vi "AlliGator Send Plots to Image Profile Window.vi"(7 "Image Control Refnum":T2, 8 "error in (no error)":errorcluster, 9 "Fit Parameter":T1, 11 "AlliGator IV DVR in":refnum<data-value>) -> (0 "error out":errorcluster, 3 "AlliGator IV DVR out":refnum<data-value>)   [LabVIEW 2021, in "AlliGator Image Profile Window.lvlib"]
doc: "Computes plots and send them to the Profile Window."
uses:
  AlliGator Image Profile Window.lvlib
  AlliGator Internal Variables v2.ctl
  <vilib>/vision/Image Controls.llb/IMAQ Image.ctl
  AlliGator Gate Image Set.ctl
  AlliGator FLI Dataset Type.ctl
  AlliGator Data Series Type.ctl
  AlliGator Dataset Channel.ctl
  AlliGator Gate Arithmetic.ctl
  AlliGator Displayed Image.ctl
  Image/Named ROI Description.ctl
  AlliGator Decay Metadata v3.ctl
  AlliGator Decay Background Subtraction Info.ctl
  AlliGator Baseline Subtraction Method.ctl
  Graphs/XY Graph/XY Graph Plot Shift Parameters.ctl
  Graphs/XY Graph/XY Graph Plot Shift Method.ctl
  AlliGator Decay Extrapolation Parameters.ctl
  Phasor/Calibration Phasor (m, phi).ctl
  Phasor/Phasor Reference Series.ctl
  Phasor/Phasor Calibration Map v2.ctl
  Phasor/Phasor (g, s).ctl
  AlliGator Raw Phasor Plot Data v4.ctl
  Phasor/Phasor Standard Deviation Options.ctl
  AlliGator Phasor Multi-Harmonic Data.ctl
  Phasor/Phasor Harmonic Data.ctl
  AlliGator Decay Fit Options & Parameters v2.ctl
  Fits/IRF(X)PSED/Decay Fit Options v2.ctl
  Fits/Decay Convolution/Decay Model.ctl
  Fits/Residual Type.ctl
  Fits/IRF(X)PSED/Fit Weights Type.ctl
  Fits/Non-linear Fitting Method v2.ctl
  Fits/Fit Calculation Method.ctl
  Fits/Non-linear Fitting Algorithm.ctl
  AlliGator Decay Fit Parameter Constraints 2.ctl
  Fits/IRF(X)PSED/Decay Fit Parameters In List.ctl
  Fits/IRF(X)PSED/MLE Baseline Offset Type.ctl
  AlliGator Decay Preprocessing Parameters.ctl
  Fits/IRF(X)PSED/Decay Fit Parameters & Derived Quantities List.ctl
  Image/Image Control Refnum.ctl
  AlliGator Variables List.ctl
  AlliGator Source Image Profile Window Event Refnum.ctl
  AlliGator Image Profile Plot Data.ctl
  Graphs/XY Graph/XY Plot Data.ctl
  AlliGator Settings List.ctl
  Image/Box Profile Type.ctl
  AlliGator Image Profile Average Intensity Type.ctl
  AlliGator Image Profile Intensity Type.ctl
  Image/Image ROI Type.ctl
  Phasor/Phasor Ratio Type.ctl
  AlliGator Phasor Ratio Color-Coded Quantity.ctl
  Variant/Variant to Data/Variant to Boolean.vi
  Variant/Variant to Data/Variant to DBL.vi
  Variant/Variant to Data/Variant to U16.vi
  AlliGator Globals, Variables & Constants.lvlib
  Graphs/XY Graph/XY Graph Add-Ons.lvlib
  Image/Image.lvlib
  AlliGator Settings.lvlib
  Variant/Variant to Data/Variant to Data.lvlib
  AlliGator Decay Fit Parameter Map.lvlib
  Phasor/Phasor.lvlib
  AlliGator Phasor Ratio.lvlib
  Arrays/Arrays.lvlib
  Error/Error.lvlib
  AlliGator Internal Variables.lvlib
  AlliGator Files.lvlib
  AlliGator Phasor Graph.lvlib
  AlliGator Decay Preprocessing.lvlib
  AlliGator Phasor Plot.lvlib
  AlliGator Source Image.lvlib
  Fits/Fits.lvlib
  AlliGator Decay Fit.lvlib
  AlliGator Dual-Channel Datasets.lvlib
panel:
  # "see the AlliGator License on the block diagram (Ctrl+E or Window:Show Block Diagram)"
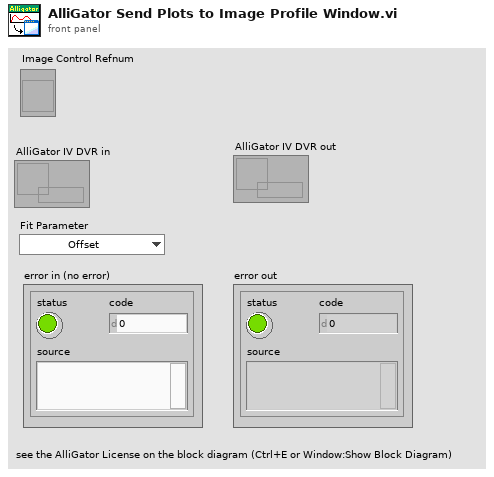
[diagram p1: front panel]
types:
  T1 = typedef "Fits.lvlib/Decay Fit Parameters & Derived Quantities List.ctl" = enum16{"Offset", "Baseline", "A_1", "tau_1", "A_2", "tau_2", "<tau>_a", "f1_a", "f2_a", "<tau>_i", "f1_i", "f2_i", "-", "R^2", "Chi^2"}
  T2 = typedef "Image.lvlib/Image Control Refnum.ctl" = refnum<vi>
  T3 = typedef "AlliGator Globals, Variables & Constants.lvlib/AlliGator Variables List.ctl" = enum16{"---- GUI ----", "Initialization Status", "State Indicators Refnum", "Original AlliGator Menu Items", "Current Action Loop State", "Script in progress", "Playback", "Loop Playback", "Search ROI Used", "Search ROI", "Decay Graph Max Legend Size", "Intensity Graph Max Legend Size", "Decay Statistics Graph Max Legend Size", "Phasor Graph Max Legend Size", "Phasor Ratio Graph Max Legend Size", "Lifetime Graph Max Legend Size", "---- Files ----", "Export Dataset Frames as Individual Files", "Show Batch Export Help Balloons", "Frames in Dataset", "ptu File Frame Start Indices", "Current Frame in Dataset", "Current Frame Timestamp", "------ Python Plugins ------", "Python Plugins Information", "Python Session", "Valid Python Session?", "---- Source Image ----", "Dataset Loaded", "Dataset Metadata", "Dataset Channel", "Dataset Data Description", "Background Dataset Metadata", "Background Dataset Channel", "Background Dataset Data Description", "Background File Subtraction", "Background File Path", "Background File Pile-up Correction", "Background File Pixel Well Capacity", "Background File Scaling Factor", "Source Image ROIs", "Current Source Image ROI", "Source Image ROI Event Refnum", "X_Source Image Display Range", "X_Source Image Palette Information", "Source Image Palette List", "Source Image Scale", "Current Dataset Load Settings", "Source Image:ROI Overlay Color", "---- Image Profile Window ----", "Image Profile:Overlay ROI in Source Image", "Image Profile Window Event Refnum", "Image Profile:IntensityType", "Image Profile:Intensity Average Type", "Image Profile:Intensity-weighted SDV", "Image Profile:Box Profile Type", "Image Profile Window Open", "Image Profile:Plotted Fit Parameter", "X_Type of Displayed Image", "X_Time Gate Slider", "Dataset Path", "Source Image Overlay to Erase", "Is Displayed Image Accumulated", "White Light Image Modified", "Mask Image Modified", "Macrotime Gate Separation", "------ Phasor Graph -------", "Phasor Graph:Show Line", "---- Phasor Plot ---", "Phasor Plot Parameters Changed", "FLI Dataset Modified since last Phasor Plot Calculation", "Phasor Harmonics Data", "Selected Phasor Harmonics", "Phasor Harmonic Manager Event Refnum", "Phasor Plot ROIs", "Current Phasor Plot ROI", "Phasor Plot ROI Event Refnum", "Phasor Plot Image Reference Points", "Phasor Plot Computed", "Phasor Plot Palette Information", "Phasor Plot Palette List", "Phasor Ratio Palette Information", "Phasor Ratio Palette List", "Phasor Image Scale", "Phasor Plot Image Overlay to Erase", "Phasor Plot Image Elements to Update", "Current Phasor Plot Calculation Parameters", "Current Phasor Calibration Options", "Reset Cumulated Phasor Plot", "Phasor Ratio Reference 1", "Phasor Ratio Lifetime Reference 1", "Phasor Ratio Reference 1 Frequency", "Phasor Ratio Reference 2", "Phasor Ratio Lifetime Reference 2", "Phasor Ratio Reference 2 Frequency", "---- Decay Analysis ----", "Number of Selected Decays to Fit", "LS Fit Results", "LAR Fit Results", "BS Fit Results", "Last Decay Max - Min", "Best Fit Parameters", "Best Fit Parameter Names", "Actual Size X", "Actual Size Y", "Binning X", "Binning Y", "Actual # Gates", "Dataset Number", "Gates to...", "Gates Skipped", "Gates to keep", "Gate Step", "Gate Separation", "Reversed Gates", "Pile-up Correction", "Pixel Well Capacity", "Background Subtracted", "Background Subtraction Method", "Background Definition Range", "Background File (deprecated)", "Number of Dataset Accumulated", "Array of Accumulated Dataset Paths", "Do Averaged Datasets", "Destination File Path", "Process Plot Target", "Use 1/D as Phasor Frequency", "---- Decay Fit Parameter Map -----", "Decay Fit Parameter Map Palette Information", "Decay Fit Parameter Map Palette List", "Local Decay Graph Window Event Refnum", "------- Local Decay Window ---------", "Use normalized IRF for convolution", "----- Miscellaneous ----", "Skippable Dialog Windows Status"}
  T4 = typedef "AlliGator Image Profile Window.lvlib/AlliGator Image Profile Intensity Type.ctl" = enum16{"Raw Data", "Displayed Image", "Background-subtracted"}
  T5 = typedef "AlliGator Image Profile Window.lvlib/AlliGator Image Profile Average Intensity Type.ctl" = enum16{"Integrated Intensity", "Average Intensity", "Intensity-weighted Average Intensity"}
  T6 = typedef "Image.lvlib/Box Profile Type.ctl" = enum16{"Full Width", "Half Width"}
  T7 = typedef "AlliGator Settings.lvlib/AlliGator Settings List.ctl" = enum16{"GUI:Visible Settings Tab", "GUI:Last Run Version", "Source Image:Use Image Histogram for Contrast", "Source Image:Low Count Pixels Rejection Options", "Source Image:High Count Pixels Rejection Options", "Source Image:Use Image Brightness", "Source Image:Blend Overlay with Image Background", "Source Image:Use Fixed ROI Diameter", "Source Image:ROI Diameter", "Source Image:ROI Center Color", "Source Image:Peak Threshold", "Source Image:Intensity Threshold", "Source Image:Image Binning Options", "Source Image:Image Smoothing Options", "Source Image:Image Histogram Active", "Source Image:Invert Binary Mask", "Source Image:Hot Pixel Removal", "Source Image:Overlay Analyzed ROI Center", "Source Image:Auto-Adjust Contrast", "Source Image:Histogram Lower Percentile", "Source Image:Histogram Upper Percentile", "Source Image:Save Source Image", "Source Image:Scale Bar Options", "Source Image:Image Resolution (Pixel Size)", "Source Image:Flatfield Correction", "Source Image:Show Dead Left Columns Correction", "Source Image:Dead Left Columns Correction", "Source Image:Image Pre-Processing Operations Order", "Data Information:Gate Width", "Data Information:Nanotime Gate Separation", "Data Information:Macrotime Gate Separation", "Data Information:Gate Step", "Data Information:# Gates", "Data Information:Gate Image Exposure", "Data Information:Gate Image Integration", "Data Information:Gates to Skip", "Data Information:Gates to Keep", "Data Information:Define Gates to", "Data Information:Channel Name", "Data Information:Available Channel Names", "Data Information:Channel Arithmetic", "Data Information:Background File Subtraction", "Data Information:Background File", "Data Information:Background Scaling Factor", "Data Information:Background Pile-up Correction", "Data Information:Background Pixel Well Capacity", "Data Information:Laser Period", "Data Information:SYNC Period", "Data Information:Pile-up Correction", "Data Information:Pixel Well Capacity", "Data Information:Dataset Scaling Factor", "Fluorescence Decay_Decay Pre-Processing:Reverse Gates", "Fluorescence Decay_Decay Pre-Processing:Verbose Decay Pre-Processing", "Fluorescence Decay_Decay Pre-Processing:Use Decay Pre-Processing", "Fluorescence Decay_Decay Pre-Processing:Background Subtraction", "Fluorescence Decay_Decay Pre-Processing:Background Definition Range", "Fluorescence Decay_Decay Pre-Processing:Baseline Subtraction Method", "Fluorescence Decay_Decay Pre-Processing:Decay Pre-Processing Operations Order", "Fluorescence Decay_Decay Pre-Processing:Smoothing Parameter", "Fluorescence Decay_Decay Pre-Processing:Shift Decay", "Fluorescence Decay_Decay Pre-Processing:Decay Shift Parameters", "Fluorescence Decay_Decay Pre-Processing:Fold Decay", "Fluorescence Decay_Decay Pre-Processing:# Folds", "Fluorescence Decay_Decay Pre-Processing:1-Normalize Decay", "Fluorescence Decay_Decay Pre-Processing:[0-1]-Normalize Decay", "Fluorescence Decay_Decay Pre-Processing:Smoothen Decay", "Fluorescence Decay_Decay Pre-Processing:Extrapolate Decay", "Fluorescence Decay_Decay Pre-Processing:Use Periodicity", "Fluorescence Decay_Decay Pre-Processing:Use Cursors", "Fluorescence Decay_Decay Pre-Processing:Tail Fraction", "Fluorescence Decay_Decay Pre-Processing:Head Fraction", "Fluorescence Decay_Decay Pre-Processing:Additional Points", "Fluorescence Decay_Decay Pre-Processing:Straighten Decay", "Fluorescence Decay_Decay Pre-Processing:Constant Background", "Fluorescence Decay_Decay Pre-Processing:Pixel-Normalize Decay", "Fluorescence Decay_Advanced Analysis:Extract IRF instead of Decay", "Fluorescence Decay_Advanced Analysis:IRF Extraction Options", "Fluorescence Decay_Advanced Analysis:IRF Optimization Options", "Fluorescence Decay_Advanced Analysis:Square Pulse Options", "Fluorescence Decay_Advanced Analysis:IRF Order", "Fluorescence Decay_Advanced Analysis:IRF Time Constants", "Fluorescence Decay_Advanced Analysis:Wavelet Analysis Options", "Fluorescence Decay_Advanced Analysis:Average Lifetime Options", "Fluorescence Decay_Fit Options:Fit Options", "Fluorescence Decay_Fit Options:Use Legacy Fitting Approach", "Fluorescence Decay_Fit Options:Use Data Information Laser Period", "Fluorescence Decay_Fit Parameters:Displayed Fit Parameters", "Fluorescence Decay_Fit Parameters:Fit Parameter Constraints", "Fluorescence Decay_Fit Parameters:Export Tabulated Results", "Fluorescence Decay_Fit Parameters:MLE Baseline Offset Type", "Fluorescence Decay_Fit Parameters:MLE Baseline Offset", "Fluorescence Decay_Fit Parameters:Guess Parameter Names", "Fluorescence Decay_Fit Parameters:Guess Parameter Values", "Fluorescence Decay_Fit Parameters:Guess Parameters Options", "Fluorescence Decay_Styles:Show Last Decay Only", "Fluorescence Decay_Styles:Decay Graph Color Array", "Fluorescence Decay:Decay Graph Active", "Fluorescence Decay Statistics:Min Peak Value", "Fluorescence Decay Statistics:Reject Low Decay Peak Pixels", "Fluorescence Decay Statistics:Reject High Decay Peak Pixels", "Fluorescence Decay Statistics:Max Peak Value", "Time Traces:Use File Timestamp", "Time Traces:Time Step", "Time Traces:Use Intensity Correction File", "Time Traces:Intensity Correction File", "Phasor Plot:Phasor Plot Smoothing Options", "Phasor Plot:Phasor Plot Size", "Phasor Plot:Phasor Plot Graphics Options", "Phasor Plot:Cumulative Phasor Plot", "Phasor Plot:Use Phasor Brightness", "Phasor Plot:Blend Overlay with Phasor Background", "Phasor Plot:Save Phasor Plot", "Phasor Plot:Show References", "Phasor Plot:Phasor Ratio Decay Range", "Phasor Plot:Exponential Fading", "Phasor Plot:Phasor Ratio Reference Colors", "Phasor Plot:Reference Radius", "Phasor Plot:Show Color Map Vertices", "Phasor Plot:Phasor Plot Active", "Phasor Plot:Phasor Ratio Color Map Type", "Phasor Plot:Phasor Ratio Color Map", "Phasor Plot:Phasor Ratio Display Range", "Phasor Plot:Selected Image ROI(s)", "Phasor Plot:All Image ROIs", "Phasor Plot:Selected Phasor Plot ROI(s)", "Phasor Plot:All Phasor Plot ROIs", "Phasor Plot:Phasor Ratio Color-Coded Quantity", "Phasor Plot:Store Phasor Harmonics", "Phasor Plot:Draw Reference Segment", "Phasor Plot:User-Defined Quantity", "Phasor Graph:Phasor Frequency", "Phasor Graph:Phasor Ratio Type", "Phasor Graph:Pixel-level Phasor Computation", "Phasor Graph:Save Phasor Graph", "Phasor Graph:Phasor Graph Active", "Phasor Graph:Phasor SDV Options", "Phasor Calibration:Use Backup Calibration if needed", "Phasor Graph:Define Shortest Lifetime as", "Phasor Calibration:Backup Calibration Type", "Phasor Calibration:Calibration Type", "Phasor Calibration:Calibration Lifetime", "Phasor Calibration:Calibration Map Algorithm", "Single-Exponential Phasor Locus (SEPL):Gate Parameters", "Single-Exponential Phasor Locus (SEPL):User-defined Gate", "Single-Exponential Phasor Locus (SEPL):User-defined IRF", "Single-Exponential Phasor Locus (SEPL):Phasor Parameters", "Single-Exponential Phasor Locus (SEPL):Decay & IRF Parameters", "Single-Exponential Phasor Locus (SEPL):Display Parameters", "Lifetime Analysis:Decay Analysis Parameters", "Lifetime Analysis:Lifetime Map Active", "Plugins:Python Settings", "Miscellaneous:Verbose Mode", "Miscellaneous:Beep after Script", "Miscellaneous:Saved Image File Format", "Miscellaneous:Exported Gate Image Settings", "Miscellaneous:Include Loading in Timing", "Miscellaneous:Verbose Settings Mode", "Miscellaneous:Histogram Options", "Miscellaneous:Beep on Error", "Miscellaneous:# Logical Processors Used", "Miscellaneous:ROI Description Max Characters", "Miscellaneous:Verbose Error Mode", "Miscellaneous:Transparent Mask Color"}
  T8 = typedef "AlliGator Image Profile Window.lvlib/AlliGator Source Image Profile Window Event Refnum.ctl" = refnum<user-event>
  T9 = typedef "AlliGator Phasor Ratio.lvlib/AlliGator Phasor Ratio Color-Coded Quantity.ctl" = enum16{"Phasor Ratio (f1 or a1)", "Average Lifetime (<tau>_i or <tau>_a))", "User-Defined Quantity"}
  T10 = typedef "Image.lvlib/Image ROI Type.ctl" = enum16{"No Selection", "Point", "Line", "Rectangle", "Oval", "Polygon", "Freehand Region", "Annulus", "Unused2", "Unused3", "Broken Line", "Freehand Line", "Rotated Rectangle"}
  T11 = typedef "Phasor.lvlib/Phasor Ratio Type.ctl" = enum32{"Intensity-weighted", "Amplitude-weighted"}
  T12 = typedef "AlliGator Internal Variables.lvlib/AlliGator Internal Variables v2.ctl" = cluster{"Displayed Image":T13, "White Light Image":T13, "Mask Image":T13, "ROI Mask Image":T13, "Current Dataset Images 1":T14, "Background Dataset Images 1":T14, "Current Dataset Images 2":T14, "Background Dataset Images 2":T14, "Current Dataset Arithmetic Images":T14, "Accumulated Dataset Images 1":T14, "Accumulated Dataset Images 2":T14, "Accumulated Dataset Arithmetic Images":T14, "Phasor Plot Image":T13, "Decay Fit Parameter Map Image":T13, "Single Data Point Path":path, "White Light Image Path":path, "Mask Image Path":path, "Time-Series Folder":path, "[Time-Series Paths]":path[], "Current Dataset":i32, "Single Dataset Type":T15, "Current Folder":string, "AlliGator Data Series Type":T16, "# Datasets":i32, "Dual-Channel Dataset":bool, "Selected Channel Name":string, "Dataset Channel":T17, "Channel Arithmetic":T18, "Dual-Channel Background Dataset":bool, "Background Channel":T17, "Dual-Channel Accumulated Dataset":bool, "Start Time":dbl, "[Time-Series Timestamps]":dbl[], "[Intensity Corrections]":dbl[], "Time Series Script":bool, "Type of Displayed Image":T19, "Gate Image Slide":u16, "# Gates":i32, "ROIs":T20[], "ROI Decay":cluster{"t Array":dbl[], "I Array":dbl[]}, "Valid Decay":bool, "Decay  Metadata":T22, "Reference Decay Plot Name":string, "Reference Decay":cluster{"t Array":dbl[], "I Array":dbl[]}, "Decay Shift Plot":cluster{"Time Stamps":dbl[], "Decay Shifts":dbl[]}, "[Decays Max Values]":sgl[], "[Decays Min Values]":sgl[], "Calibration Phasor":T28, "Calibration Phasor Series":T29, "Phasor Calibration Map":T30, "Calibration Map MD5 Digest":string, "Last Raw Phasor":T31, "Last Calibrated Phasor":T31, "Last Calibrated Phasor SDV":T31, "Phasor Graph:Phasor Plot":cluster{"g Array":dbl[], "s Array":dbl[]}, "Phasor Graph:Phasor SDV Plot":cluster{"g Array":dbl[], "s Array":dbl[]}, "[Phasor Graph:Raw Phasor Plots]":T32[], "Phasor Plot locked to Ref 1":i32, "[Phasor Plot(s) locked to Ref 1]":i32[], "[Phasor Plot(s) locked to Ref 2]":i32[], "[Pixel Phasors]":T31[], "[[Sum Image]]":dbl[][], "[[CSG Phasors]]":csg[][], "[[Valid Pixel?]]":bool[][], "I/m/phi Dataset":cluster{"I/m/phi Dataset?":bool, "Base Frequency":dbl[unit], "Harmonic Orders":u8[]}, "Multi Phasor Plot Data":T34, "Decay Fit Options & Parameters":T36, "Fit Options: Decay Preprocessing Parameters":T47, "Fit Options: Reference Decay":cluster{"t Array":dbl[], "I Array":dbl[]}, "Is Full Image Parameters Map":bool, "Is Single-Pixels Parameters Map":bool, "NLSF Parameters Map X Resolution":i32, "NLSF Parameters Map Y Resolution":i32, "[Single Decay Fit Parameters]":dbl[], "Fit Model":T38, "[[Multiple Decays Fit Parameters]]":dbl[][], "[[Multiple Decays Fit Parameter SDVs]]":dbl[][], "[[IRFs]]":dbl[][], "IRF Array Time Axis":dbl[], "Decay Array Time Axis":dbl[], "[Decay Fit Parameter Names]":T1[], "[[Phasor Ratios]]":dbl[][], "[[Average Lifetimes]]":dbl[][], "Amplitude Weighted Average Lifetime":bool, "[Decay Sum]":dbl[], "[[User-defined Quantities]]":dbl[][], "User-defined Quantity":string}
  T13 = typedef "IMAQ Image.ctl" = refnum<image>
  T14 = typedef "AlliGator Internal Variables.lvlib/AlliGator Gate Image Set.ctl" = cluster{"SGL Image Max":T13, "SGL Image Sum":T13, "SGL Gate Images":T13[], "SGL Image Min":T13}
  T15 = typedef "AlliGator Files.lvlib/AlliGator FLI Dataset Type.ctl" = enum16{"HDF5 FLI Dataset", "Gate Image Folder", ".sdt FLI Dataset (Becker & Hickl)", ".ptu FLI Dataset (PicoQuant)", "SS1 FLI Dataset", "SS2 FLI Dataset", "I/m/phi Dataset", ".bin FLI Dataset (PicoQuant Binned)", ".bin FLI Dataset (Piccolo Binned)"}
  T16 = typedef "AlliGator Files.lvlib/AlliGator Data Series Type.ctl" = enum16{"Not a Supported Series", "Gate Images Folder Series", "SwissSPAD 2 Dataset Series", "B&H FLI Dataset Series", "PicoQuant PTU FLI Dataset Series", "PicoQuant BIN FLI Dataset Series", "Piccolo hist BIN FLI Dataset Series", "HDF5 FLI Dataset Series"}
  T17 = typedef "AlliGator Dual-Channel Datasets.lvlib/AlliGator Dataset Channel.ctl" = enum16{"G2", "INT"}
  T18 = typedef "AlliGator Settings.lvlib/AlliGator Gate Arithmetic.ctl" = enum16{"None", "INT-G2", "G2/INT*<INT>", "(1 - G2/INT)*<INT>"}
  T19 = typedef "AlliGator Source Image.lvlib/AlliGator Displayed Image.ctl" = enum16{"Single Gate", "Sum of All Gates", "Max of All Gates", "Min of All Gates", "-", "White Ligth Image", "Mask Image"}
  T20 = typedef "Image.lvlib/Named ROI Description.ctl" = cluster{"ROI Descriptor":T21, "ROI Name":string, "Overlay Color":u32}
  T21 = typedef "ROI Descriptor" = cluster{"Global Rectangle":i32[], "Contours":cluster{"ID":enum32{"External", "Internal"}, "Type":u32, "Coordinates":i32[]}[]}
  T22 = typedef "AlliGator Phasor Graph.lvlib/AlliGator Decay Metadata v3.ctl" = cluster{"ROI Descriptor":T21, "ROI Center":cluster{"X":i32, "Y":i32}, "Decay Background Subtraction Info":T23, "Decay Reverted":bool, "Decay Smoothened":bool, "Decay Straightened":bool, "Fitted Tau (Decay Straightening)":dbl, "Decay Shift Parameters":T25, "Decay Shifted":bool, "Decay Extrapolated":bool, "Decay Extrapolation Parameters":T27, "Decay Normalized":bool, "Fold Decay":bool, "# Folds":u32}
  T23 = typedef "AlliGator Decay Analysis.lvlib/AlliGator Decay Preprocessing.lvlib/AlliGator Decay Background Subtraction Info.ctl" = cluster{"Laser Period":dbl[unit], "Gate Duration":dbl[unit], "Baseline Subtraction Method":T24, "Background Definition Range":cluster{"Min Gate":dbl[unit], "Max Gate":dbl[unit]}, "Total Intensity w/o Bkgd Subtraction":dbl, "Bkgd-subtracted Intensity (exp)":dbl, "# Data Points":i32, "Background/Gate":dbl, "Fitted Lifetime":dbl[unit], "Bkgd-subtracted Intensity (theo)":dbl}
  T24 = typedef "AlliGator Decay Analysis.lvlib/AlliGator Decay Preprocessing.lvlib/AlliGator Baseline Subtraction Method.ctl" = enum16{"Mean", "Min", "Square Gated Single-Exponential", "File", "Constant"}
  T25 = typedef "XY Graph Add-Ons.lvlib/XY Graph Plot Shift Parameters.ctl" = cluster{"Type":T26, "Shift":dbl[unit], "Threshold":dbl, "Rotate":bool}
  T26 = typedef "XY Graph Add-Ons.lvlib/XY Graph Plot Shift Method.ctl" = enum16{"Default", "CFD", "Threshold", "Cross-Correlation"}
  T27 = typedef "AlliGator Decay Analysis.lvlib/AlliGator Decay Preprocessing.lvlib/AlliGator Decay Extrapolation Parameters.ctl" = cluster{"Additional Points":u32, "Head Fraction":dbl, "Fitted Tau":dbl, "Use Periodicity":bool, "Use Cursors":bool, "Tail Fraction":dbl}
  T28 = typedef "Phasor.lvlib/Calibration Phasor (m, phi).ctl" = cluster{"m":dbl, "phi":dbl, "Phasor Frequency":dbl[unit], "Reference Lifetime":dbl[unit]}
  T29 = typedef "Phasor.lvlib/Phasor Reference Series.ctl" = cluster{"m Array":dbl[], "phi Array":dbl[], "Phasor Frequency":dbl[unit], "Calibration Lifetime":dbl[unit]}
  T30 = typedef "Phasor.lvlib/Phasor Calibration Map v2.ctl" = cluster{"Phasor Frequency":dbl[unit], "Calibration Lifetime":dbl[unit], "ROI Centers":cluster{"X":i32, "Y":i32}[], "ROI Descriptors":T21[], "Map Resolution X":i32, "Map Resolution Y":i32, "z Array":cdb[]}
  T31 = typedef "Phasor.lvlib/Phasor (g, s).ctl" = cluster{"g":dbl, "s":dbl}
  T32 = typedef "AlliGator Phasor Graph.lvlib/AlliGator Raw Phasor Plot Data v4.ctl" = cluster{"Phasor Plot Name":string, "Raw Phasor Plot":T31[], "Phasor Frequency":dbl[unit], "[Decay Metadata]":T22[], "Raw Phasor Plot SDV":T31[], "Phasor SDV Options":T33, "[Calibration Phasor]":T28[]}
  T33 = typedef "Phasor.lvlib/Phasor Standard Deviation Options.ctl" = cluster{"Compute Estimated SDV":bool, "# Replicas":u32, "Use Estimated Average Phasor":bool}
  T34 = typedef "AlliGator Phasor Plot.lvlib/AlliGator Phasor Multi-Harmonic Data.ctl" = cluster{"Base Frequency":dbl[unit], "# Harmonics":u8, "Harmonic Orders":u8[], "Phasor Plot Settings Checksum":u64, "Phasor Harmonic Data Array":T35[]}
  T35 = typedef "Phasor.lvlib/Phasor Harmonic Data.ctl" = cluster{"Phasor Harmonic Name":string, "Phasor Plot Settings Checksum":u64, "Phasor Frequency":dbl[unit], "Base Frequency":dbl[unit], "Harmonic Order":u8, "Phasor Plot Parameters":string, "Phasor Array [[CSG]]":csg[][], "Dataset File Path":path}
  T36 = typedef "AlliGator Decay Fit Parameter Map.lvlib/AlliGator Decay Fit Options & Parameters v2.ctl" = cluster{"SYNC Period":dbl[unit], "Fit Options":T37, "Fit Parameter Constraints":T44[], "MLE Baseline Offset":dbl, "MLE Baseline Offset Type":T46}
  T37 = typedef "Fits.lvlib/Decay Fit Options v2.ctl" = cluster{"Show Fit Residuals":bool, "Fit Model":T38, "Residual Type":T39, "Max Decay Percentile":dbl, "Min Decay Percentile":dbl, "Show Full Decay":bool, "Weights":T40, "Fitting Method":T41, "Compute Parameter Uncertainties":bool, "Periodic Boundaries":bool, "Model Calculation":T42, "Period":dbl[unit], "Termination Criteria":cluster{"Max Iterations":i32, "Max Function Calls":i32, "Max Time":dbl[unit], "Function Tolerance":dbl, "Parameter Tolerance":dbl, "Gradient Tolerance":dbl, "Min Lambda":dbl, "Max Lambda":dbl, "Initial Tick Count":u32}, "Offset Resolution":dbl[unit], "Use Local IRF":bool, "Fitting Algorithm":T43}
  T38 = typedef "Fits.lvlib/Decay Model.ctl" = enum16{"1-Exponential", "2-Exponentials"}
  T39 = typedef "Fits.lvlib/Residual Type.ctl" = enum16{"Standard", "Normalized", "Reduced"}
  T40 = typedef "Fits.lvlib/Fit Weights Type.ctl" = enum16{"Unweighted", "1/Variance", "Best of All"}
  T41 = typedef "Fits.lvlib/Non-linear Fitting Method v2.ctl" = enum16{"Least Square", "Least Absolute Residual", "Bisquare", "MLE", "-", "Best of All"}
  T42 = typedef "Fits.lvlib/Fit Calculation Method.ctl" = enum16{"Simulation", "Convolution", "Integration"}
  T43 = typedef "Fits.lvlib/Non-linear Fitting Algorithm.ctl" = enum16{"Levenberg-Marquardt", "Trust-Region Dogleg"}
  T44 = typedef "AlliGator Decay Analysis.lvlib/AlliGator Decay Fit.lvlib/AlliGator Decay Fit Parameter Constraints 2.ctl" = cluster{"Fit Parameter":T45, "Min Value":dbl, "Max Value":dbl, "Global":bool, "Used":bool}
  T45 = typedef "Fits.lvlib/Decay Fit Parameters In List.ctl" = enum16{"Offset", "Baseline", "A_1", "tau_1", "A_2", "tau_2"}
  T46 = typedef "Fits.lvlib/MLE Baseline Offset Type.ctl" = enum32{"Absolute", "Percentage"}
  T47 = typedef "AlliGator Decay Analysis.lvlib/AlliGator Decay Preprocessing.lvlib/AlliGator Decay Preprocessing Parameters.ctl" = cluster{"Background Subtraction":bool, "Straighten Decay":bool, "Reverse Gates":bool, "1-Normalized Decay":bool, "Smoothen Decay":bool, "Smoothing Parameter":dbl, "Shift Decay":bool, "Decay Shift Parameters":T25, "Extrapolate Decay":bool, "Additional Points":u32, "Head Fraction":dbl, "Pixel-Normalize Decay":bool, "Use Periodicity":bool, "Use Cursors":bool, "Tail Fraction":dbl, "Use Decay Pre-Processing":bool, "Fold Decay":bool, "# Folds":u32, "[0-1]-Normalized Decay":bool}
  T48 = cluster{"Global Rectangle":i32[], "Contours":cluster{"Contour Type":u32, "ROI Type":u32, "Points":i32[]}[]}
  T49 = cluster{"Contour Type":u32, "ROI Type":u32, "Points":i32[]}[]
  T50 = cluster{"Contour Type":u32, "ROI Type":u32, "Points":i32[]}
  T51 = typedef "AlliGator Image Profile Window.lvlib/AlliGator Image Profile Plot Data.ctl" = cluster{"Plot Name":string, "Plot":T52}
  T52 = typedef "XY Graph Add-Ons.lvlib/XY Plot Data.ctl" = cluster{"X Array":dbl[], "Y Array":dbl[]}
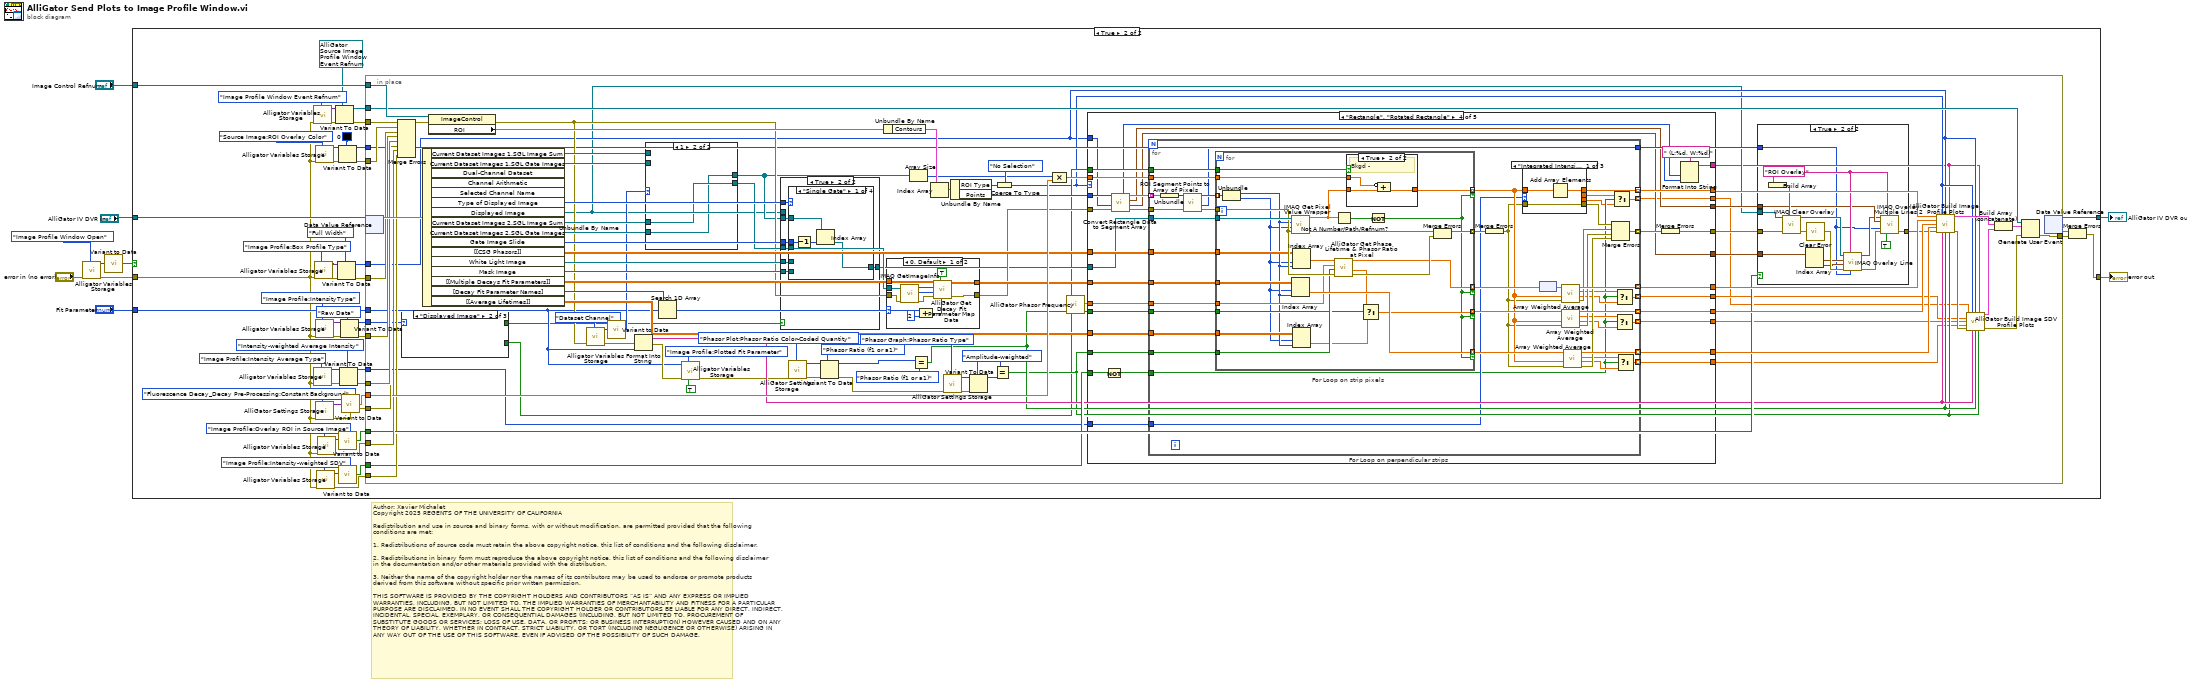
[diagram p0: block diagram]
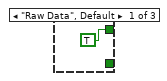
[diagram p3: hidden frame]
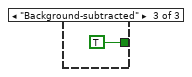
[diagram p4: hidden frame]
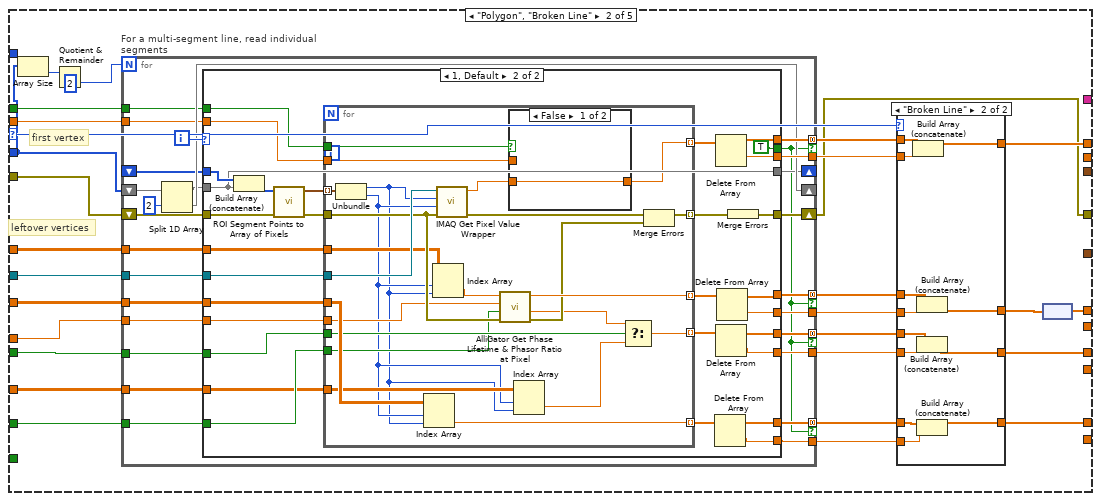
[diagram p13: hidden frame]
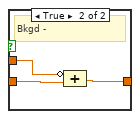
[diagram p16: hidden frame]
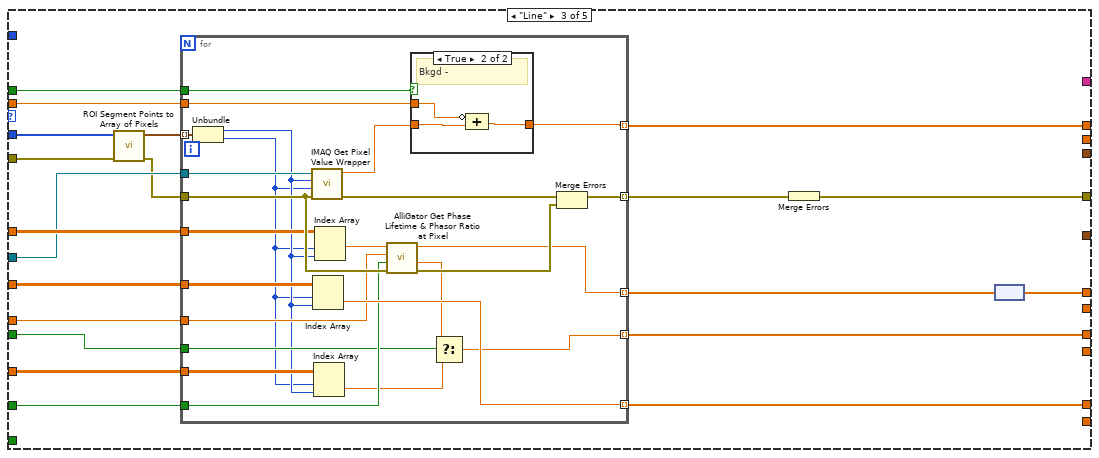
[diagram p17: hidden frame]
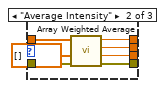
[diagram p19: hidden frame]
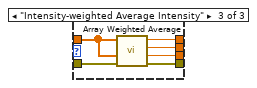
[diagram p20: hidden frame]
diagram:
  # "Author: Xavier Michalet\nCopyright 2025 REGENTS OF THE UNIVERSITY OF CALIFORNIA\n\nRedistribution and use in source and binary forms, with or without modification, are permitted provided that the following conditions are met:\n\n1. Redistributions of source code must retain the above copyright notice, this list of conditions and the following disclaimer.\n\n2. Redistributions in binary form must reproduce the above copyright notice, this list of conditions and the following disclaimer in the documentation and/or other materials provided with the distribution.\n\n3. Neither the name of the copyright holder nor the names of its contributors may be used to endorse or promote products derived from this software without specific prior written permission.\n\nTHIS SOFTWARE IS PROVIDED BY THE COPYRIGHT HOLDERS AND CONTRIBUTORS “AS IS” AND ANY EXPRESS OR IMPLIED WARRANTIES, INCLUDING, BUT NOT LIMITED TO, THE IMPLIED WARRANTIES OF MERCHANTABILITY AND FITNESS FOR A PARTICULAR PURPOSE ARE DISCLAIMED. IN NO EVENT SHALL THE COPYRIGHT HOLDER OR CONTRIBUTORS BE LIABLE FOR ANY DIRECT, INDIRECT, INCIDENTAL, SPECIAL, EXEMPLARY, OR CONSEQUENTIAL DAMAGES (INCLUDING, BUT NOT LIMITED TO, PROCUREMENT OF SUBSTITUTE GOODS OR SERVICES; LOSS OF USE, DATA, OR PROFITS; OR BUSINESS INTERRUPTION) HOWEVER CAUSED AND ON ANY THEORY OF LIABILITY, WHETHER IN CONTRACT, STRICT LIABILITY, OR TORT (INCLUDING NEGLIGENCE OR OTHERWISE) ARISING IN ANY WAY OUT OF THE USE OF THIS SOFTWARE, EVEN IF ADVISED OF THE POSSIBILITY OF SUCH DAMAGE."
  n1 = call "Alligator Variables Storage.vi"("AlliGator Variable"=AlliGator_Variables_List."Image Profile Window Open" ("Alligator Variable"), "Error In"="error in (no error)") -> ("Error Out"=w2:errorcluster, "Data out"=w5:variant)  [unwired: 7 in, 1 out]
  n2 = call-poly "Variant to Data.vi"("Variant"=w5) -> ("Value"=w1:bool)  [unwired: 8 in]
  n3 = case shown="True" w1 {
    tunnel: "AlliGator IV DVR in" -> [w12 w62]
    tunnel: [w12 w61] -> w9
    tunnel: "Image Control Refnum" -> [_ w60]
    tunnel: [w11 w52] -> w7
    tunnel: "Fit Parameter" -> [_ w50]
    tunnel: w2 -> [w11 w23]
    frame False {
    }
    frame True {
      n4 = call "Alligator Variables Storage.vi"("AlliGator Variable"=AlliGator_Variables_List."Image Profile Window Event Refnum" ("Alligator Variable"), "Error In"=w23) -> ("Error Out"=w58:errorcluster, "Data out"=w56:variant)  [unwired: 7 in, 1 out]
      n5 = call "Alligator Variables Storage.vi"("AlliGator Variable"=AlliGator_Variables_List."Image Profile:Intensity Average Type" ("Alligator Variable"), "Error In"=w23) -> ("Error Out"=w18:errorcluster, "Data out"=w19:variant)  [unwired: 7 in, 1 out]
      n6 = call "Alligator Variables Storage.vi"("AlliGator Variable"=AlliGator_Variables_List."Image Profile:Box Profile Type" ("Alligator Variable"), "Error In"=w23) -> ("Error Out"=w42:errorcluster, "Data out"=w43:variant)  [unwired: 7 in, 1 out]
      n7 = call "Alligator Variables Storage.vi"("AlliGator Variable"=AlliGator_Variables_List."Source Image:ROI Overlay Color" ("Alligator Variable"), "Error In"=w23) -> ("Error Out"=w32:errorcluster, "Data out"=w30:variant)  [unwired: 7 in, 1 out]
      n8 = call "Alligator Variables Storage.vi"("AlliGator Variable"=AlliGator_Variables_List."Image Profile:IntensityType" ("Alligator Variable"), "Error In"=w23) -> ("Error Out"=w22:errorcluster, "Data out"=w20:variant)  [unwired: 7 in, 1 out]
      n9 = call "AlliGator Settings Storage.vi"("AlliGator Settings List"=AlliGator_Settings_List."Fluorescence Decay_Decay Pre-Processing:Constant Background", "Error In"=w23) -> ("Error Out"=w48:errorcluster, "Variant Data out"=w46:variant)  [unwired: 8 in]
      n10 = call "Alligator Variables Storage.vi"("AlliGator Variable"=AlliGator_Variables_List."Image Profile:Intensity-weighted SDV" ("Alligator Variable"), "Error In"=w23) -> ("Error Out"=w26:errorcluster, "Data out"=w25:variant)  [unwired: 7 in, 1 out]
      n11 = call "Alligator Variables Storage.vi"("AlliGator Variable"=AlliGator_Variables_List."Image Profile:Overlay ROI in Source Image" ("Alligator Variable"), "Error In"=w23) -> ("Error Out"=w36:errorcluster, "Data out"=w37:variant)  [unwired: 7 in, 1 out]
      n12 = Variant To Data(error in=w58, type=T8 refnum ("Profile Window Event"), Variant=w56) -> (data=w54:T8, error out=w57:errorcluster)
      n13 = Variant To Data(error in=w42, type=Box_Profile_Type."Full Width" ("Box Profile Type"), Variant=w43) -> (data=w40:T6, error out=w39:errorcluster)
      n14 = call-poly "Variant to Data.vi"("Variant"=w25) -> ("Value"=w27:bool)  [unwired: 8 in]
      n15 = Variant To Data(error in=w32, type=u32 0, Variant=w30) -> (data=w28:u32, error out=w31:errorcluster)
      n16 = call-poly "Variant to Data.vi"("Variant"=w37) -> ("Value"=w34:bool)  [unwired: 8 in]
      n17 = Variant To Data(error in=w18, type=AlliGator_Image_Profile_Average_Intensity_Type."Intensity-weighted Average Intensity" ("Image Profile Average Intenisty Type"), Variant=w19) -> (data=w13:T5, error out=w17:errorcluster)
      n18 = Variant To Data(error in=w22, type=AlliGator_Image_Profile_Intensity_Type."Raw Data" ("Image Profile Intensity Type"), Variant=w20) -> (data=w15:T4, error out=w21:errorcluster)
      n19 = call-poly "Variant to Data.vi"("Variant"=w46) -> ("Value"=w45:dbl)  [unwired: 8 in]
      n20 = in-place {
        in-place-border: w60 -> [w155]
        in-place-border: w57 -> [w154]
        in-place-border: w54 -> [w153]
        in-place-border: w50 -> [w73]
        in-place-border: w21 -> [w151]
        in-place-border: w17 -> [w150]
        in-place-border: w48 -> [w149]
        in-place-border: w45 -> [w148]
        in-place-border: w40 -> [w66]
        in-place-border: w39 -> [w147]
        in-place-border: w36 -> [w104]
        in-place-border: [w97] -> w35
        in-place-border: w34 -> [w94]
        in-place-border: w31 -> [w93]
        in-place-border: w28 -> [w92]
        in-place-border: w26 -> [w88]
        in-place-border: w27 -> [w87]
        in-place-border: w15 -> [w71]
        in-place-border: w13 -> [w68]
        w123 = Phasor_Ratio_Type."Amplitude-weighted" ("Phasor Ratio Type")
        n21 = in-place-dvr #1(w62) -> (w156:T12)  [unwired: 1 out]
        n22 = Merge Errors(w154, w93, w147, w151, w150, w149, w104, w88) -> (w152:errorcluster)
        n23 = case shown="\"Displayed Image\"" w71 {
          tunnel: [TRUE ("Get(F)/Set") _ _] -> w70
          tunnel: [_ _ TRUE ("Get(F)/Set")] -> w69
          frame "Raw Data", Default {
          }
          frame "Displayed Image" {
          }
          frame "Background-subtracted" {
          }
        }
        n24 = Unbundle By Name(w156) -> ("Current Dataset Images 1.SGL Image Sum"=w126:T13, "Current Dataset Images 1.SGL Gate Images"=w125:T13[], "Type of Displayed Image"=w138:T19, "Displayed Image"=w65:T13, "Current Dataset Images 2.SGL Image Sum"=w127:T13, "Current Dataset Images 2.SGL Gate Images"=w128:T13[], "Gate Image Slide"=w137:u16, "[[CSG Phasors]]"=w139:csg[][], "White Light Image"=w136:T13, "Mask Image"=w135:T13, "[[Multiple Decays Fit Parameters]]"=w132:dbl[][], "[Decay Fit Parameter Names]"=w131:T1[], "[[Average Lifetimes]]"=w113:dbl[][])  [unwired: 3 out]
        n25 = property class="ImageControl"(reference=w155, error in=w152) -> (error out=w110:errorcluster, "ROI"=w146:T48)  [unwired: 1 out]
        n26 = call "Alligator Variables Storage.vi"("AlliGator Variable"=AlliGator_Variables_List."Dataset Channel" ("Alligator Variable"), "Error In"=w110) -> ("Error Out"=w109:errorcluster, "Data out"=w112:variant)  [unwired: 7 in, 1 out]
        n27 = call-poly "Variant to Data.vi"("Variant"=w112) -> ("U16 Value"=w108:u16)  [unwired: 8 in]
        n28 = Format Into String(error in=w109, w73) -> (resulting string=w85:string, error out=w75:errorcluster)  [unwired: 2 in]
        n29 = case shown="1" w108 {
          tunnel: [w177 w179] -> w129
          tunnel: w127 -> [_ w179]
          tunnel: [w176 w178] -> w107
          tunnel: w128 -> [_ w178]
          tunnel: w126 -> [w177 _]
          tunnel: w125 -> [w176 _]
          frame 0, Default {
          }
          frame 1 {
          }
        }
        n30 = Search 1D Array(1D array=w131, element=w73) -> (index of element=w134:i32)  [unwired: 1 in]
        n31 = call "Alligator Variables Storage.vi"("Get(F)/Set"=TRUE, "AlliGator Variable"=AlliGator_Variables_List."Image Profile:Plotted Fit Parameter" ("Alligator Variable"), "Error In"=w75, "Data in"=w73) -> ("Error Out"=w74:errorcluster)  [unwired: 5 in, 2 out]
        n32 = case shown="True" w70 {
          tunnel: w65 -> [w193 _]
          tunnel: [w193 w198] -> w91
          tunnel: w138 -> [_ w200]
          tunnel: w129 -> [_ w199]
          tunnel: w137 -> [_ w197]
          tunnel: w107 -> [_ w196]
          tunnel: w136 -> [_ w195]
          tunnel: w135 -> [_ w194]
          frame False {
          }
          frame True {
            n33 = case shown="\"Single Gate\"" w200 {
              tunnel: w199 -> [_ _ _ w207]
              tunnel: [w201 w205 w206 w207] -> w198
              tunnel: w197 -> [w203 _ _ _]
              tunnel: w196 -> [w204 _ _ _]
              tunnel: w195 -> [_ w205 _ _]
              tunnel: w194 -> [_ _ w206 _]
              frame "Single Gate" {
                n34 = Decrement(x=w203) -> (x-1=w202:u16)
                n35 = Index Array(array=w204, index=w202) -> (element=w201:T13)
              }
              frame "White Ligth Image" {
              }
              frame "Mask Image" {
              }
              frame "Sum of All Gates", Default {
              }
            }
          }
        }
        n36 = call "AlliGator Settings Storage.vi"("AlliGator Settings List"=AlliGator_Settings_List."Phasor Plot:Phasor Ratio Color-Coded Quantity", "Error In"=w74) -> ("Error Out"=w119:errorcluster, "Variant Data out"=w117:variant)  [unwired: 8 in]
        n37 = Variant To Data(error in=w119, type=AlliGator_Phasor_Ratio_Color-Coded_Quantity."Phasor Ratio (f1 or a1)" ("Displayed Quantity"), Variant=w117) -> (data=w115:T9, error out=w118:errorcluster)
        n38 = Unbundle By Name(w146) -> ("Contours"=w145:T49)
        n39 = case shown="0, Default" w134 {
          selector: w134 -> [w186 _]
          tunnel: w129 -> [w185 _]
          tunnel: w132 -> [w184 _]
          tunnel: [w181 _] -> w133
          tunnel: w110 -> [w183 w192]
          tunnel: [w180 w192] -> w99
          frame 0, Default {
            n40 = call "IMAQ GetImageInfo"("error in (no error)"=w183, "Image"=w185) -> ("error out"=w191:errorcluster, "Y Resolution"=w190:i32, "X Resolution"=w189:i32)  [unwired: 2 in, 5 out]
            n41 = Compound Arithmetic op=ADD(w186, 2 ("value")) -> (w188:i32)
            n42 = call "AlliGator Get Decay Fit Parameter Map Data.vi"("Map index"=w188, "Compute Decay Fit Parameter Map"=TRUE, "Error In"=w191, "Y Resolution"=w190, "X Resolution"=w189, "Multiple Decays Fit Parameters"=w184) -> ("Error Out"=w180:errorcluster, "Map Data (V x H)"=w181:dbl[][])  [unwired: 3 in, 1 out]
          }
          frame ..-1 {
          }
        }
        n43 = Array Size(array=w107) -> (size(s)=w105:i32)
        n44 = Equal?(x=w115, y=AlliGator_Phasor_Ratio_Color-Coded_Quantity."Phasor Ratio (f1 or a1)") -> (x = y?=w84:bool)
        n45 = Index Array(array=w145) -> (element=w144:T50)  [unwired: 1 in]
        n46 = call "AlliGator Settings Storage.vi"("AlliGator Settings List"=AlliGator_Settings_List."Phasor Graph:Phasor Ratio Type", "Error In"=w118) -> ("Error Out"=w121:errorcluster, "Variant Data out"=w122:variant)  [unwired: 8 in]
        n47 = Unbundle By Name(w144) -> ("ROI Type"=w142:u32, "Points"=w143:i32[])
        n48 = Variant To Data(error in=w121, type=w123, Variant=w122) -> (data=w124:T11)  [unwired: 1 out]
        n49 = Equal?(x=w123, y=w124) -> (x = y?=w83:bool)
        n50 = Coerce To Type(0:w142, 1:Image_ROI_Type."No Selection" ("ROI Type")) -> (2:w67:T10)
        n51 = Compound Arithmetic op=MULTIPLY(w105, w148) -> (w106:dbl)
        n52 = call "AlliGator Phasor Frequency.vi"() -> ("Phasor Frequency"=w140:dbl[unit])
        n53 = case shown="\"Rectangle\", \"Rotated Rectangle\"" w67 {
          selector: w67 -> [_ w214 _ _ _]
          tunnel: w99 -> [w208 w237 w356 w406 w520]
          tunnel: [w208 w210 w342 w410 w514] -> w96
          tunnel: w143 -> [_ w209 w341 w421 w533]
          tunnel: [_ w231 w355 w418 w532] -> w103
          tunnel: w139 -> [_ w230 w360 w420 w529]
          tunnel: w140 -> [_ w229 w358 w419 w528]
          tunnel: [_ w213 w345 w409 w517] -> w102
          tunnel: w91 -> [_ w225 w354 w417 w527]
          tunnel: [_ w222 w352 w416 w526] -> w101
          tunnel: w133 -> [_ w221 w351 w415 w525]
          tunnel: [_ w219 w350 w414 w524] -> w100
          tunnel: w83 -> [_ w217 w349 w413 w523]
          tunnel: w113 -> [_ w216 w348 w412 w522]
          tunnel: w84 -> [_ w215 w347 w411 w521]
          tunnel: w69 -> [_ w212 w344 w404 w516]
          tunnel: w106 -> [_ w211 w343 w403 w515]
          tunnel: w66 -> [_ _ _ w402 _]
          tunnel: [_ _ _ w390 _] -> w90
          tunnel: [_ _ _ w399 _] -> w63
          tunnel: [_ _ _ w391 _] -> w89
          tunnel: w87 -> [_ _ _ w397 _]
          tunnel: [_ _ _ w395 _] -> w82
          tunnel: [_ _ _ w394 _] -> w81
          tunnel: [_ _ _ w393 _] -> w80
          tunnel: w68 -> [_ _ _ w392 _]
          tunnel: [_ _ _ w389 _] -> w64
          frame "No Selection", Default {
          }
          frame "Polygon", "Broken Line" {
            # "leftover vertices"
            # "first vertex"
            n54 = Array Size(array=w209) -> (size(s)=w236:i32)
            n55 = Quotient & Remainder(x=w236, y=2) -> (floor(x/y)=w235:i32)  [unwired: 1 out]
            n56 = for "For a multi-segment line, read individual segments" {
              N: w235 -> [_]
              shift-right: [w279] -> w210
              shift-left: w237 -> [w280]
              tunnel: [w277] -> w233 mode=concatenating if=w260
              tunnel: [w276] -> w232
              shift-right: [w272] -> _
              shift-left: w209 -> [w275]
              shift-right: [w270] -> _
              shift-left: _ -> [w269]
              tunnel: w230 -> [w268]
              tunnel: w229 -> [w267]
              tunnel: [w266] -> w228 mode=concatenating if=w260
              tunnel: [w265] -> w226
              tunnel: w225 -> [w278]
              tunnel: [w264] -> w224 mode=concatenating if=w260
              tunnel: [w263] -> w223
              tunnel: w221 -> [w262]
              tunnel: [w261] -> w220 mode=concatenating if=w260
              tunnel: [w259] -> w218
              tunnel: w217 -> [w258]
              tunnel: w216 -> [w257]
              tunnel: w215 -> [w256]
              tunnel: w212 -> [w255]
              tunnel: w211 -> [w254]
              i -> [w273]
              n57 = Split 1D Array(array=w275, index=2) -> (first subarray=w271:i32[], second subarray=w272:i32[])
              n58 = case shown="1, Default" w273 {
                tunnel: w280 -> [w281 w298]
                tunnel: [w281 w308] -> w279
                tunnel: w278 -> [_ w299]
                tunnel: [_ w312] -> w277
                tunnel: [_ w311] -> w276
                tunnel: w271 -> [w282 w285]
                tunnel: [w282 w285] -> w270
                tunnel: w269 -> [_ w286]
                tunnel: [_ TRUE] -> w260
                tunnel: w268 -> [_ w306]
                tunnel: w267 -> [_ w305]
                tunnel: [_ w303] -> w266
                tunnel: [_ w302] -> w265
                tunnel: [_ w295] -> w264
                tunnel: [_ w294] -> w263
                tunnel: w262 -> [_ w293]
                tunnel: [_ w291] -> w261
                tunnel: [_ w290] -> w259
                tunnel: w258 -> [_ w289]
                tunnel: w257 -> [_ w287]
                tunnel: w256 -> [_ w288]
                tunnel: w255 -> [_ w284]
                tunnel: w254 -> [_ w283]
                frame 0 {
                  # "preserves the previous point"
                }
                frame 1, Default {
                  n59 = Build Array (concatenate)(w286, w285) -> (w309:i32[])
                  n60 = call "ROI Segment Points to Array of Pixels.vi"("error in (no error)"=w298, "Segment ROI Points"=w309) -> ("Error Out"=w297:errorcluster, "Pixels of the Segment"=w307:cluster{"X":i32, "Y":i32}[])  [unwired: 7 in, 1 out]
                  n61 = for {
                    tunnel: w307 -> [w336] mode=indexing
                    tunnel: w306 -> [w326]
                    tunnel: w305 -> [w325]
                    tunnel: [w335] -> w304 mode=indexing
                    tunnel: [w332] -> w301 mode=indexing
                    tunnel: [w315] -> w300 mode=indexing
                    tunnel: w297 -> [w330]
                    tunnel: w299 -> [w333]
                    tunnel: [w322] -> w296 mode=indexing
                    tunnel: w293 -> [w329]
                    tunnel: [w328] -> w292 mode=indexing
                    tunnel: w289 -> [w320]
                    tunnel: w287 -> [w319]
                    tunnel: w288 -> [w321]
                    tunnel: w284 -> [w314]
                    tunnel: w283 -> [w313]
                    n62 = Unbundle(w336) -> ("X"=w317:i32, "Y"=w318:i32)
                    n63 = Index Array(array=w329, index (row)=w318, index (col)=w317) -> (element=w328:dbl)
                    n64 = Index Array(array=w326, index (row)=w318, index (col)=w317) -> (element=w327:csg)
                    n65 = call "IMAQ Get Pixel Value Wrapper.vi"("Error In"=w330, "Y Coordinate"=w318, "X Coordinate"=w317, "Image"=w333) -> ("Error Out"=w334:errorcluster, "Pixel Value"=w316:sgl)  [unwired: 5 in, 1 out]
                    n66 = call "AlliGator Get Phase Lifetime & Phasor Ratio at Pixel.vi"("error in (no error)"=w330, "Intensity (F)/Amplitude (T) weighted"=w320, "Phasor Frequency"=w325, "Phasor"=w327) -> ("error out"=w331:errorcluster, "Phasor/Amplitude Ratio"=w323:dbl, "Phase Lifetime"=w335:dbl[unit])  [unwired: 4 in, 1 out]
                    n67 = case shown="False" w314 {
                      tunnel: w316 -> [w337 w340]
                      tunnel: [w337 w339] -> w315
                      tunnel: w313 -> [_ w338]
                      frame False {
                      }
                      frame True {
                        # "Bkgd -"
                        n68 = Compound Arithmetic op=ADD(invert w338, w340) -> (w339:dbl)
                      }
                    }
                    n69 = Index Array(array=w319, index (row)=w318, index (col)=w317) -> (element=w324:dbl)
                    n70 = Select(t=w323, s=w321, f=w324) -> (s? t:f=w322:dbl)
                    n71 = Merge Errors(w334, w331) -> (w332:errorcluster)
                  }
                  n72 = Delete From Array(array=w292) -> (deleted portion=w290:dbl, array with subset deleted=w291:dbl[])  [unwired: 2 in]
                  n73 = Delete From Array(array=w300) -> (deleted portion=w311:dbl, array with subset deleted=w312:dbl[])  [unwired: 2 in]
                  n74 = Delete From Array(array=w296) -> (deleted portion=w294:dbl, array with subset deleted=w295:dbl[])  [unwired: 2 in]
                  n75 = Delete From Array(array=w304) -> (deleted portion=w302:dbl[unit], array with subset deleted=w303:dbl[unit][])  [unwired: 2 in]
                  n76 = Merge Errors(w301) -> (w308:errorcluster)
                }
              }
            }
            n77 = case shown="\"Broken Line\"" w214 {
              tunnel: w233 -> [w241 w253]
              tunnel: w232 -> [_ w252]
              tunnel: [w241 w251] -> w231
              tunnel: w228 -> [w240 w250]
              tunnel: [w240 w249] -> w227
              tunnel: w226 -> [_ w248]
              tunnel: w224 -> [w239 w247]
              tunnel: w223 -> [_ w246]
              tunnel: [w239 w245] -> w222
              tunnel: w220 -> [w238 w244]
              tunnel: [w238 w243] -> w219
              tunnel: w218 -> [_ w242]
              frame "Polygon", Default {
              }
              frame "Broken Line" {
                n78 = Build Array (concatenate)(w253, w252) -> (w251:dbl[])
                n79 = Build Array (concatenate)(w250, w248) -> (w249:dbl[unit][])
                n80 = Build Array (concatenate)(w247, w246) -> (w245:dbl[])
                n81 = Build Array (concatenate)(w244, w242) -> (w243:dbl[])
              }
            }
            n82 = node(w227) -> (w213:dbl[])
          }
          frame "Line" {
            n83 = call "ROI Segment Points to Array of Pixels.vi"("error in (no error)"=w356, "Segment ROI Points"=w341) -> ("Error Out"=w353:errorcluster, "Pixels of the Segment"=w359:cluster{"X":i32, "Y":i32}[])  [unwired: 7 in, 1 out]
            n84 = for {
              tunnel: w360 -> [w375]
              tunnel: w359 -> [w384] mode=indexing
              tunnel: w358 -> [w373]
              tunnel: [w376] -> w346 mode=indexing
              tunnel: w354 -> [w383]
              tunnel: w353 -> [w378]
              tunnel: [w381] -> w357 mode=indexing
              tunnel: [w363] -> w355 mode=indexing
              tunnel: [w368] -> w352 mode=indexing
              tunnel: w351 -> [w380]
              tunnel: [w379] -> w350 mode=indexing
              tunnel: w349 -> [w372]
              tunnel: w348 -> [w367]
              tunnel: w347 -> [w371]
              tunnel: w344 -> [w362]
              tunnel: w343 -> [w361]
              n85 = Unbundle(w384) -> ("X"=w366:i32, "Y"=w365:i32)
              n86 = call "IMAQ Get Pixel Value Wrapper.vi"("Error In"=w378, "Y Coordinate"=w365, "X Coordinate"=w366, "Image"=w383) -> ("Error Out"=w382:errorcluster, "Pixel Value"=w364:sgl)  [unwired: 5 in, 1 out]
              n87 = Index Array(array=w380, index (row)=w365, index (col)=w366) -> (element=w379:dbl)
              n88 = Index Array(array=w367, index (row)=w365, index (col)=w366) -> (element=w370:dbl)
              n89 = Index Array(array=w375, index (row)=w365, index (col)=w366) -> (element=w374:csg)
              n90 = call "AlliGator Get Phase Lifetime & Phasor Ratio at Pixel.vi"("error in (no error)"=w378, "Intensity (F)/Amplitude (T) weighted"=w372, "Phasor Frequency"=w373, "Phasor"=w374) -> ("error out"=w377:errorcluster, "Phasor/Amplitude Ratio"=w369:dbl, "Phase Lifetime"=w376:dbl[unit])  [unwired: 4 in, 1 out]
              n91 = case shown="True" w362 {
                tunnel: w364 -> [w385 w388]
                tunnel: [w385 w387] -> w363
                tunnel: w361 -> [_ w386]
                frame False {
                }
                frame True {
                  # "Bkgd -"
                  n92 = Compound Arithmetic op=ADD(invert w386, w388) -> (w387:dbl)
                }
              }
              n93 = Select(t=w369, s=w371, f=w370) -> (s? t:f=w368:dbl)
              n94 = Merge Errors(w382, w377) -> (w381:errorcluster)
            }
            n95 = Merge Errors(w357) -> (w342:errorcluster)
            n96 = node(w346) -> (w345:dbl[])
          }
          frame "Rectangle", "Rotated Rectangle" {
            n97 = Not(x=w397) -> (.not. x?=w396:bool)
            n98 = call "Convert Rectangle Data to Segment Array.vi"("Error In"=w406, "Box Profile Type"=w402, "(Rotated) Rectangle Data"=w421) -> ("Error Out"=w405:errorcluster, "Median End Points"=w390:cluster{"X":dbl, "Y":dbl}[], "Rectangle End Points"=w391:cluster{"X":dbl, "Y":dbl}[], "Rectange Profile Segments"=w408:cluster{"Segment ROI Points":i32[]}[], "Number of Points"=w398:i32)  [unwired: 4 in]
            n99 = for "For Loop on perpendicular strips" {
              tunnel: w408 -> [w466] mode=indexing
              tunnel: w420 -> [w465]
              tunnel: w419 -> [w463]
              tunnel: [w449] -> w407 mode=indexing
              tunnel: w405 -> [w461]
              tunnel: [w439] -> w418 mode=indexing
              tunnel: w417 -> [w460]
              tunnel: [w451] -> w416 mode=indexing
              tunnel: w415 -> [w458]
              tunnel: [w445] -> w414 mode=indexing
              tunnel: w413 -> [w457]
              tunnel: w412 -> [w456]
              tunnel: w411 -> [w455]
              tunnel: [w450] -> w409 mode=indexing
              tunnel: w404 -> [w441]
              tunnel: w403 -> [w440]
              tunnel: [w438] -> w400
              tunnel: w396 -> [w425]
              tunnel: [w431] -> w395 mode=indexing
              tunnel: [w430] -> w394 mode=indexing
              tunnel: [w429] -> w393 mode=indexing
              tunnel: w392 -> [w428]
              tunnel: [w422] -> w389 mode=indexing
              n100 = Unbundle(w466) -> ("Segment ROI Points"=w443:i32[])
              n101 = call "ROI Segment Points to Array of Pixels.vi"("error in (no error)"=w461, "Segment ROI Points"=w443) -> ("Error Out"=w459:errorcluster, "Number of Points"=w438:i32, "Pixels of the Segment"=w464:cluster{"X":i32, "Y":i32}[])  [unwired: 7 in]
              n102 = for "For Loop on strip pixels" {
                tunnel: w465 -> [w499]
                tunnel: w464 -> [w508] mode=indexing
                tunnel: w463 -> [w497]
                tunnel: [w500] -> w454 mode=indexing if=w483
                tunnel: w460 -> [w507]
                tunnel: w459 -> [w502]
                tunnel: [w505] -> w462 mode=indexing
                tunnel: [w486] -> w442 mode=indexing if=w483
                tunnel: [w492] -> w452 mode=indexing if=w483
                tunnel: w458 -> [w504]
                tunnel: [w503] -> w446 mode=indexing if=w483
                tunnel: w457 -> [w496]
                tunnel: w456 -> [w491]
                tunnel: w455 -> [w495]
                tunnel: w441 -> [w488]
                tunnel: w440 -> [w487]
                n103 = Unbundle(w508) -> ("X"=w490:i32, "Y"=w489:i32)
                n104 = call "IMAQ Get Pixel Value Wrapper.vi"("Error In"=w502, "Y Coordinate"=w489, "X Coordinate"=w490, "Image"=w507) -> ("Error Out"=w506:errorcluster, "Pixel Value"=w485:sgl)  [unwired: 5 in, 1 out]
                n105 = Index Array(array=w504, index (row)=w489, index (col)=w490) -> (element=w503:dbl)
                n106 = Index Array(array=w491, index (row)=w489, index (col)=w490) -> (element=w494:dbl)
                n107 = Index Array(array=w499, index (row)=w489, index (col)=w490) -> (element=w498:csg)
                n108 = call "AlliGator Get Phase Lifetime & Phasor Ratio at Pixel.vi"("error in (no error)"=w502, "Intensity (F)/Amplitude (T) weighted"=w496, "Phasor Frequency"=w497, "Phasor"=w498) -> ("error out"=w501:errorcluster, "Phasor/Amplitude Ratio"=w493:dbl, "Phase Lifetime"=w500:dbl[unit])  [unwired: 4 in, 1 out]
                n109 = Not A Number/Path/Refnum?(number/path/refnum=w485) -> (NaN/Path/Refnum?=w484:bool)
                n110 = case shown="True" w488 {
                  tunnel: w485 -> [w509 w512]
                  tunnel: [w509 w511] -> w486
                  tunnel: w487 -> [_ w510]
                  frame False {
                  }
                  frame True {
                    # "Bkgd -"
                    n111 = Compound Arithmetic op=ADD(invert w510, w512) -> (w511:dbl)
                  }
                }
                n112 = Select(t=w493, s=w495, f=w494) -> (s? t:f=w492:dbl)
                n113 = Not(x=w484) -> (.not. x?=w483:bool)
                n114 = Merge Errors(w506, w501) -> (w505:errorcluster)
              }
              n115 = Merge Errors(w462) -> (w427:errorcluster)
              n116 = case shown="\"Integrated Intensity\", Default" w428 {
                tunnel: w442 -> [w469 w476 w479]
                tunnel: [w468 w475 w482] -> w439
                tunnel: [_ w474 w481] -> w424
                tunnel: [_ w473 w480] -> w423
                tunnel: w427 -> [w467 w472 w478]
                tunnel: [w467 w471 w477] -> w426
                frame "Integrated Intensity", Default {
                  n117 = Add Array Elements(numeric array=w469) -> (sum=w468:dbl)
                }
                frame "Average Intensity" {
                  n118 = call "Array Weighted Average.vi"("Error In"=w472, "Weight Array"=dbl[] [], "Array"=w476) -> ("Error Out"=w471:errorcluster, "SDV (weighted)"=w473:dbl, "SDV (classic)"=w474:dbl, "Average Value (weighted)"=w475:dbl)  [unwired: 5 in]
                }
                frame "Intensity-weighted Average Intensity" {
                  n119 = call "Array Weighted Average.vi"("Error In"=w478, "Weight Array"=w479, "Array"=w479) -> ("Error Out"=w477:errorcluster, "SDV (weighted)"=w480:dbl, "SDV (classic)"=w481:dbl, "Average Value (weighted)"=w482:dbl)  [unwired: 5 in]
                }
              }
              n120 = node(w454) -> (w453:dbl[])
              n121 = call "Array Weighted Average.vi"("Error In"=w427, "Weight Array"=w442, "Array"=w453) -> ("Error Out"=w448:errorcluster, "SDV (weighted)"=w436:dbl, "SDV (classic)"=w437:dbl, "Average Value (weighted)"=w450:dbl)  [unwired: 5 in]
              n122 = call "Array Weighted Average.vi"("Error In"=w427, "Weight Array"=w442, "Array"=w452) -> ("Error Out"=w447:errorcluster, "SDV (weighted)"=w434:dbl, "SDV (classic)"=w435:dbl, "Average Value (weighted)"=w451:dbl)  [unwired: 5 in]
              n123 = call "Array Weighted Average.vi"("Error In"=w427, "Weight Array"=w442, "Array"=w446) -> ("Error Out"=w444:errorcluster, "SDV (weighted)"=w432:dbl, "SDV (classic)"=w433:dbl, "Average Value (weighted)"=w445:dbl)  [unwired: 5 in]
              n124 = Merge Errors(w426, w448, w447, w444) -> (w449:errorcluster)
              n125 = Select(t=w424, s=w425, f=w423) -> (s? t:f=w422:dbl)
              n126 = Select(t=w437, s=w425, f=w436) -> (s? t:f=w431:dbl)
              n127 = Select(t=w435, s=w425, f=w434) -> (s? t:f=w430:dbl)
              n128 = Select(t=w433, s=w425, f=w432) -> (s? t:f=w429:dbl)
            }
            n129 = Merge Errors(w407) -> (w410:errorcluster)
            n130 = Format Into String(format string=" (L:%d, W:%d)", w398, w400) -> (resulting string=w399:string)  [unwired: 2 in, 1 out]
          }
          frame "Freehand Line" {
            n131 = call "Remove Duplicate Consecutive Vertices.vi"("Error In"=w520, "Freehand Line Points (in)"=w533) -> ("Error Out"=w519:errorcluster, "Freehand Line Points (out)"=w513:i32[])  [unwired: 8 in]
            n132 = Decimate 1D Array(w513) -> (w531:i32[], w530:i32[])
            n133 = for {
              tunnel: w531 -> [w540] mode=indexing
              tunnel: [w537] -> w532 mode=indexing
              tunnel: w530 -> [w539] mode=indexing
              tunnel: w528 -> [w548]
              tunnel: [w551] -> w518 mode=indexing
              tunnel: w529 -> [w549]
              tunnel: w527 -> [w556]
              tunnel: w519 -> [w552]
              tunnel: [w555] -> w534 mode=indexing
              tunnel: [w544] -> w526 mode=indexing
              tunnel: w525 -> [w541]
              tunnel: [w554] -> w524 mode=indexing
              tunnel: w523 -> [w543]
              tunnel: w522 -> [w542]
              tunnel: w521 -> [w547]
              tunnel: w516 -> [w536]
              tunnel: w515 -> [w535]
              n134 = Index Array(array=w549, index (row)=w539, index (col)=w540) -> (element=w550:csg)
              n135 = Index Array(array=w542, index (row)=w539, index (col)=w540) -> (element=w545:dbl)
              n136 = call "IMAQ Get Pixel Value Wrapper.vi"("Error In"=w552, "Y Coordinate"=w539, "X Coordinate"=w540, "Image"=w556) -> ("Error Out"=w557:errorcluster, "Pixel Value"=w538:sgl)  [unwired: 5 in, 1 out]
              n137 = call "AlliGator Get Phase Lifetime & Phasor Ratio at Pixel.vi"("error in (no error)"=w552, "Intensity (F)/Amplitude (T) weighted"=w543, "Phasor Frequency"=w548, "Phasor"=w550) -> ("error out"=w553:errorcluster, "Phasor/Amplitude Ratio"=w546:dbl, "Phase Lifetime"=w551:dbl[unit])  [unwired: 4 in, 1 out]
              n138 = case shown="True" w536 {
                tunnel: w538 -> [w558 w561]
                tunnel: [w558 w560] -> w537
                tunnel: w535 -> [_ w559]
                frame False {
                }
                frame True {
                  # "Bkgd -"
                  n139 = Compound Arithmetic op=ADD(invert w559, w561) -> (w560:dbl)
                }
              }
              n140 = Select(t=w546, s=w547, f=w545) -> (s? t:f=w544:dbl)
              n141 = Index Array(array=w541, index (row)=w539, index (col)=w540) -> (element=w554:dbl)
              n142 = Merge Errors(w557, w553) -> (w555:errorcluster)
            }
            n143 = Merge Errors(w534) -> (w514:errorcluster)
            n144 = node(w518) -> (w517:dbl[])
          }
        }
        n145 = case shown="True" w94 {
          tunnel: w96 -> [w159 w175]
          tunnel: [w159 w169] -> w95
          tunnel: w92 -> [_ w161]
          tunnel: w90 -> [_ w164]
          tunnel: w89 -> [_ w166]
          tunnel: w65 -> [_ w160]
          frame False {
          }
          frame True {
            w167 = "ROI Overlay" ("Groups")
            n146 = Build Array(w167) -> (w173:string[])
            n147 = call "IMAQ Clear Overlay"("Groups"=w173, "error in (no error)"=w175, "Image"=w160) -> ("error out"=w174:errorcluster, "Image Out"=w172:T13)  [unwired: 7 in]
            n148 = Index Array(array=w164) -> (element #1=w163:cluster{"X":dbl, "Y":dbl}, element #2=w162:cluster{"X":dbl, "Y":dbl})  [unwired: 2 in]
            n149 = call "Clear Error.vi"("Error In"=w174) -> ("no Error Out"=w171:errorcluster)  [unwired: 8 in]
            n150 = call "IMAQ Overlay Line"("Color"=w161, "Group"=w167, "error in (no error)"=w171, "End Point"=w162, "Start Point"=w163, "Image"=w172) -> ("error out"=w170:errorcluster, "Image Out"=w165:T13)  [unwired: 4 in]
            n151 = call "IMAQ Overlay Multiple Lines 2"("Image"=w165, "Group"=w167, "Line End Points"=w166, "Color"=w161, "error in (no error)"=w170, "Maintain Width?"=TRUE) -> ("error out"=w169:errorcluster)  [unwired: 8 in, 1 out]
          }
        }
        n152 = call "AlliGator Build Image Profile Plots.vi"("Intensity"=w103, "ROI Type"=w67, "Box Profile Type"=w66, "ROI Size String"=w63, "Phase Lifetime"=w102, "Average Lifetime/Phasor Ratio"=w101, "Fit Parameter"=w100, "Error In"=w95, "Fit Parameter Name"=w85, "ratio(T)/<tau>(F)"=w84, "< t>_I (F)/<t>_A"=w83) -> ("Plot Array"=w98:T51[], "Error Out"=w86:errorcluster)  [unwired: 3 in]
        n153 = call "AlliGator Build Image SDV Profile Plots.vi"("Intensity SDV"=w64, "ROI Type"=w67, "Box Profile Type"=w66, "ROI Size String"=w63, "Phase Lifetime SDV"=w82, "Average Lifetime/Phasor Ratio SDV"=w81, "Fit Parameter SDV"=w80, "Error In"=w86, "Fit Parameter Name"=w85, "ratio(T)/<tau>(F)"=w84, "< t>_I (F)/<t>_A"=w83) -> ("Plot Array"=w78:T51[], "Error Out"=w77:errorcluster)  [unwired: 3 in]
        n154 = Build Array (concatenate)(w98, w78) -> (w79:T51[])
        n155 = Generate User Event(user event=w153, event data cluster=w79, error in=w77) -> (error out=w97:errorcluster)  [unwired: 1 in, 1 out]
        n156 = in-place-dvr #1() -> (w61:refnum<data-value>, w53:errorcluster)  [unwired: 1 in]
      }
      n157 = Merge Errors(w53, w35) -> (w52:errorcluster)
    }
  }
  "error out" <- w7
  "AlliGator IV DVR out" <- w9
